vi "Launch Filter Config View.vi"(8 "error in (no error)":errorcluster, 11 "ConsoleView in":refnum<class "ConsoleView.lvclass">) -> (0 "error out":errorcluster, 3 "ConsoleView out":refnum<class "ConsoleView.lvclass">)   [LabVIEW 2020, in "MVA Framework.lvlib" / "ConsoleView.lvlib" / "ConsoleView.lvclass"]
uses:
  ConsoleView.lvclass
  ConsoleView.lvclass/ConsoleView.ctl
  Filter ConfigurationView.vi
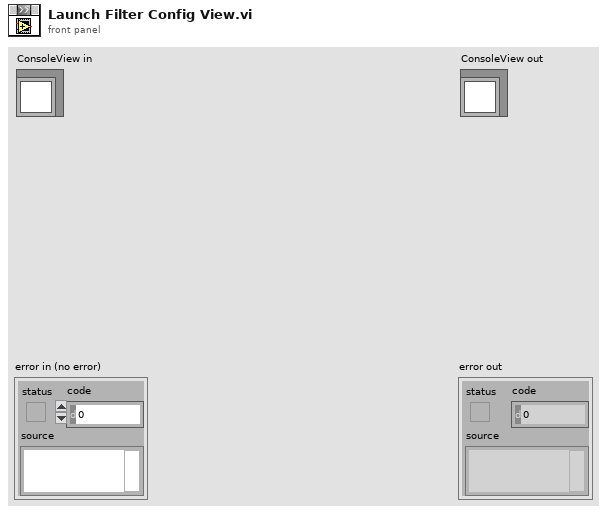
[diagram p1: front panel]
types:
  T1 = typedef "MVA Framework.lvlib/ConsoleView.lvlib/ConsoleView.lvclass/FilterConfig.ctl" = cluster{"Level Filter":cluster{"Warning":bool, "Debug":bool, "Info":bool, "Error":bool, "Critical":bool}, "Source Filter":cluster{"Source":string, "Exclude Match?":bool, "Exact Match?":bool}, "Keyword Filter":cluster{"Keywords":string[], "Exclude Match?":bool}}
  T2 = enum32{"Invalid", "Standard", "Closed", "Hidden", "Minimized", "Maximized"}
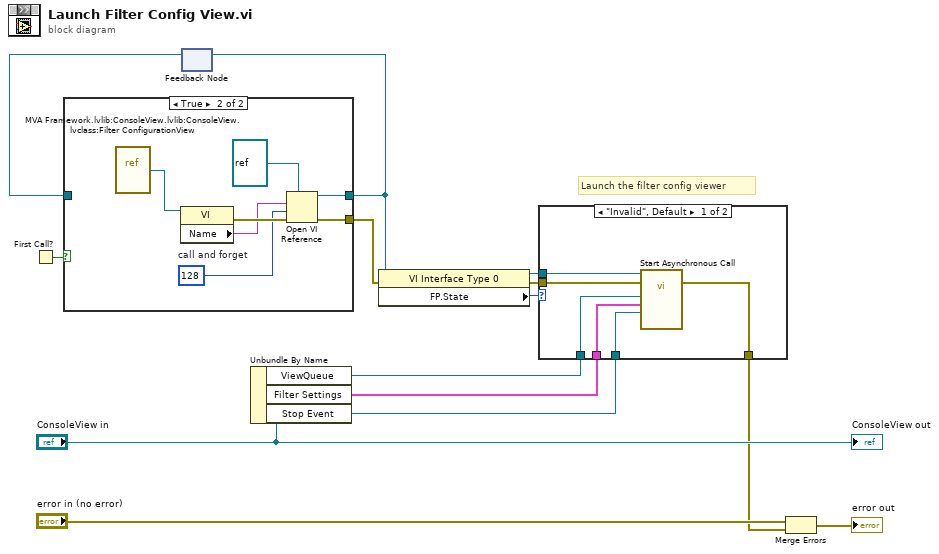
[diagram p0: block diagram]
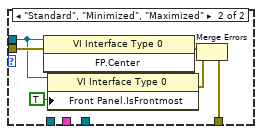
[diagram p2: hidden frame]
diagram:
  # "Launch the filter config viewer"
  n1 = First Call?() -> (First Call?: T/F=w6:bool)
  n2 = feedback #1() -> (w5:refnum<vi>)  [unwired: 1 in]
  n3 = case shown="True" w6 {
    tunnel: [_ w17] -> w12
    tunnel: [w14 w16] -> w2
    tunnel: w5 -> [w14 _]
    frame False {
    }
    frame True {
      w19 = 128  # call and forget
      n4 = vi-ref "MVA Framework.lvlib:ConsoleView.lvlib:ConsoleView.lvclass:Filter ConfigurationView.vi"() -> (w21:refnum<vi>)
      n5 = property class="VI"(reference=w21) -> (error out=w20:errorcluster, "Name"=w18:string)  [unwired: 1 in, 1 out]
      n6 = Open VI Reference(type specifier VI Refnum (for type only)=refnum<vi> refnum, vi path=w18, options=w19, error in (no error)=w20) -> (vi reference=w16:refnum<vi>, error out=w17:errorcluster)  [unwired: 2 in]
    }
  }
  n7 = feedback-in #1(w2) -> ()
  n8 = Unbundle By Name("ConsoleView in") -> ("ViewQueue"=w10:refnum<queue>, "Filter Settings"=w9:T1, "Stop Event"=w4:refnum<user-event>)
  n9 = property class="VI Interface Type 0"(reference=w2, error in=w12) -> (error out=w3:errorcluster, "FP.State"=w1:T2)  [unwired: 1 out]
  n10 = case shown="\"Invalid\", Default" w1 {
    tunnel: w10 -> [w27 _]
    tunnel: w9 -> [w26 _]
    tunnel: [w22 w29] -> w7
    tunnel: w4 -> [w25 _]
    tunnel: w3 -> [w24 w33]
    tunnel: w2 -> [w23 w31]
    frame "Invalid", Default {
      n11 = call-by-ref "Start Asynchronous Call"(reference=w23, error in=w24, "Stop Event"=w25, "Current Filter Settings"=w26, "ViewQueue"=w27) -> (error out=w22:errorcluster)  [unwired: 9 in, 1 out]
    }
    frame "Standard", "Minimized", "Maximized" {
      n12 = invoke class="VI Interface Type 0" method="FP.Center"(reference=w31, error in=w33) -> (error out=w32:errorcluster)  [unwired: 1 in, 2 out]
      n13 = property class="VI Interface Type 0"(reference=w31, "Front Panel.IsFrontmost"=TRUE ("Front Panel Window:Is Frontmost")) -> (error out=w28:errorcluster)  [unwired: 1 in, 1 out]
      n14 = Merge Errors(w32, w28) -> (w29:errorcluster)
    }
  }
  n15 = Merge Errors("error in (no error)", w7) -> (→"error out":errorcluster)
  "ConsoleView out" <- "ConsoleView in"
